vi "Lancador2.vi"() -> ()   [LabVIEW 2019]
panel:
  out "LancadorB":dbl
  out "Lancador2":dbl
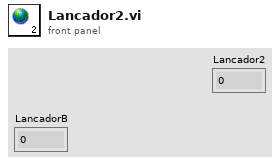
[diagram p1: front panel]
diagram:
